vi "Read All.vi"(8 "error in (no error)":errorcluster, 11 "Online_Statistic in":refnum<class "Online_Statistic.lvclass">) -> (0 "error out":errorcluster, 2 "Statistics":T1, 3 "Online_Statistic out":refnum<class "Online_Statistic.lvclass">)   [LabVIEW 2021, in "Online_Statistic.lvclass"]
uses:
  Online_Statistic.lvclass
  Online_Statistic.lvclass/Online_Statistic.ctl
  Read Cumulative_mean.vi
  Read Cumulative_mean_square .vi
  Read Cumulative_variance.vi
  Read Max.vi
  Read Min.vi
  Read Number_of_samples.vi
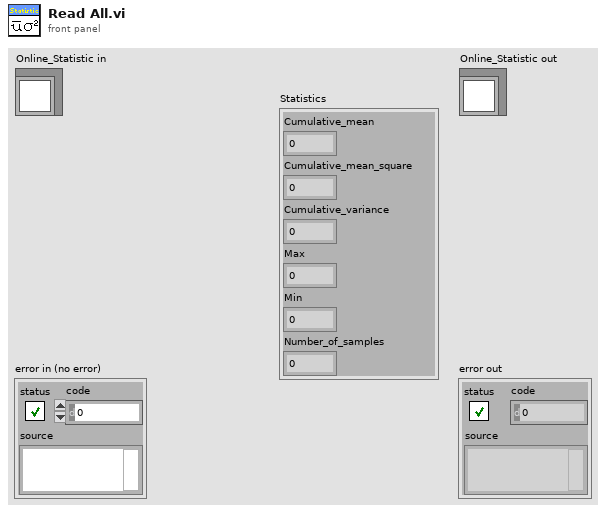
[diagram p1: front panel]
types:
  T1 = cluster{"Cumulative_mean":dbl, "Cumulative_mean_square ":dbl, "Cumulative_variance":dbl, "Max":dbl, "Min":dbl, "Number_of_samples":i32}
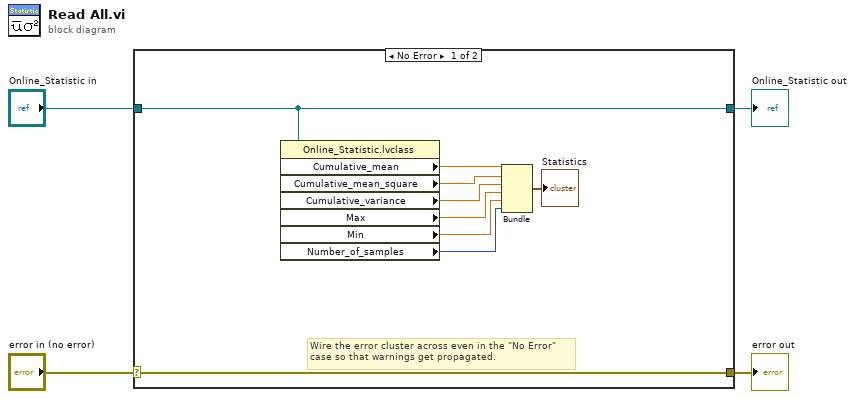
[diagram p0: block diagram]
diagram:
  n1 = case shown="No Error" "error in (no error)" {
    selector: "error in (no error)" -> [w13 w15]
    tunnel: [w13 w15] -> w3
    tunnel: [w12 w14] -> w1
    tunnel: "Online_Statistic in" -> [w12 w14]
    frame No Error {
      # "Wire the error cluster across even in the \"No Error\"\ncase so that warnings get propagated."
      n2 = property class="Online_Statistic.lvclass"(reference=w12) -> ("Cumulative_mean"=w11:dbl, "Cumulative_mean_square "=w10:dbl, "Cumulative_variance"=w9:dbl, "Max"=w8:dbl, "Min"=w7:dbl, "Number_of_samples"=w6:i32)  [unwired: 1 in, 2 out]
      n3 = Bundle("Cumulative_mean"=w11, "Cumulative_mean_square"=w10, "Cumulative_variance"=w9, "Max"=w8, "Min"=w7, "Number_of_samples"=w6) -> (→"Statistics":T1)  [unwired: 1 in]
    }
    frame Error {
    }
  }
  "error out" <- w3
  "Online_Statistic out" <- w1
